vi "Get SMO HELP.vi"(8 "error in (no error)":errorcluster, 10 "Command":string, 11 "Instrument.Framework-Template in":refnum<class "Instrument.Framework-Template.lvclass">) -> (0 "error out":errorcluster, 2 "output cluster":T1, 3 "Instrument.Framework-Template out":refnum<class "Instrument.Framework-Template.lvclass">)   [LabVIEW 2019, in "Instrument.Framework-Template.lvclass"]
uses:
  Instrument.Framework-Template.lvclass
  C:/Users/patrick/Documents/GitHub/Instrument-Framework/lvsrc/Framework/Instrument/Instrument.lvclass
  <userlib>/LevyLab/Instrument Framework/Instrument/Help/typedefs/Help--cluster.ctl
  Typedefs/Instrument.Framework-Template.PublicCommands--Enum.ctl
  <userlib>/LevyLab/Instrument Framework/Instrument Types/SCPI/Instrument.SCPI.lvclass
  <userlib>/LevyLab/Instrument Framework/Instrument/Help/Help.lvclass
  <userlib>/LevyLab/Instrument Framework/Instrument/Instrument.lvclass
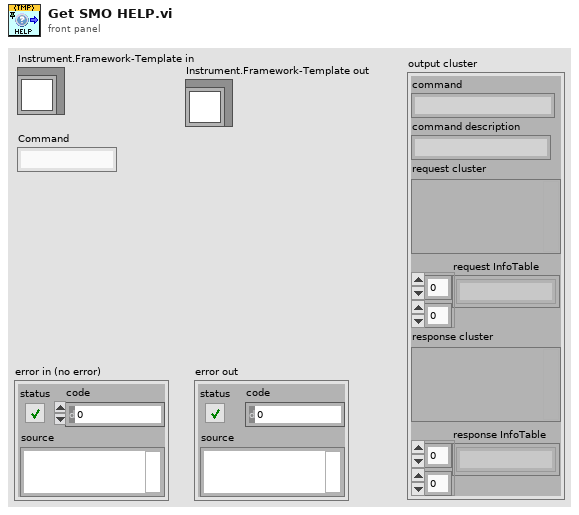
[diagram p1: front panel]
types:
  T1 = typedef "Help.lvclass/Help--cluster.ctl" = cluster{"command":string, "command description":string, "request cluster":variant, "request InfoTable":string[][], "response cluster":variant, "response InfoTable":string[][]}
  T2 = typedef "Instrument.Framework-Template.lvclass/Instrument.Framework-Template.PublicCommands--Enum.ctl" = enum16{"doSomething"}
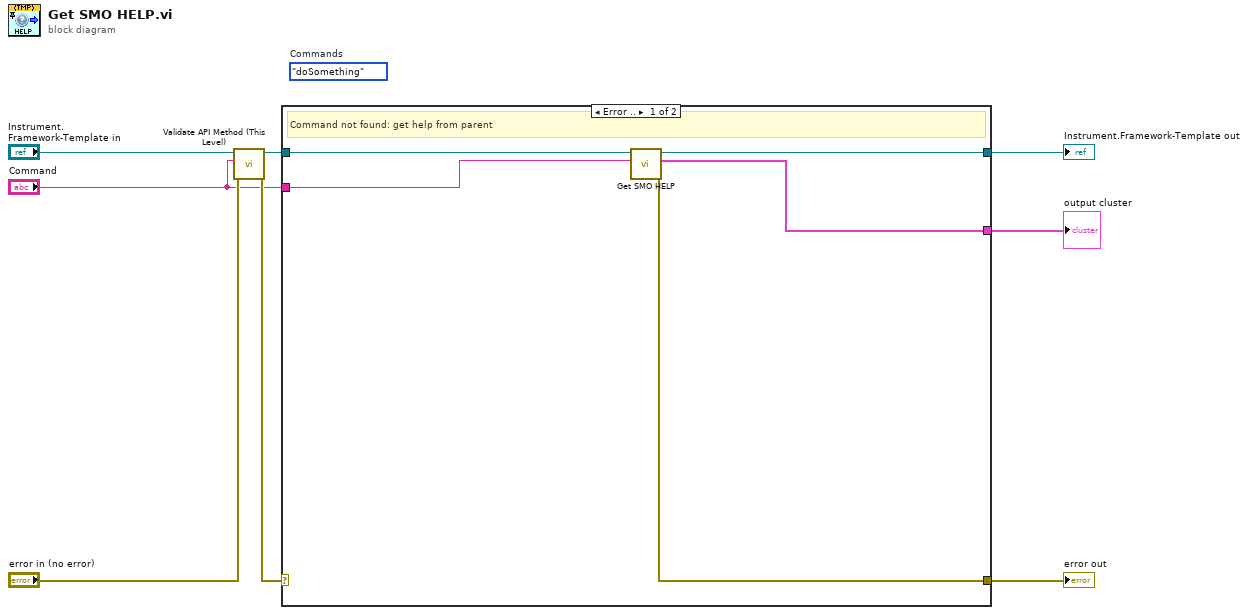
[diagram p0: block diagram]
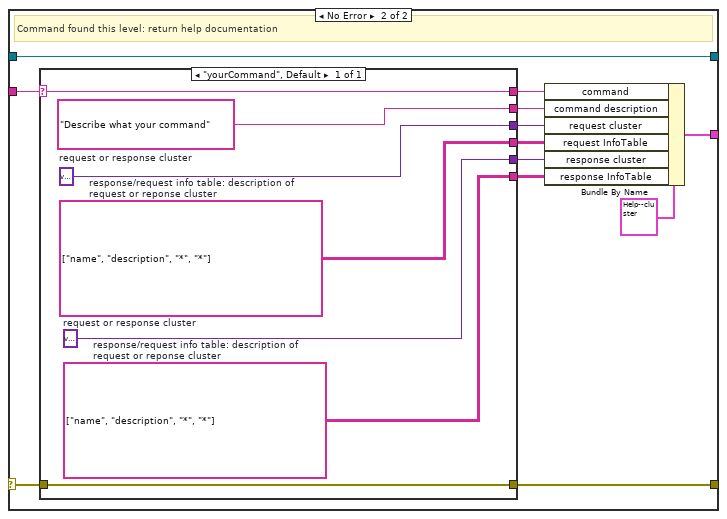
[diagram p2: hidden frame]
diagram:
  (unwired) Instrument.Framework-Template.PublicCommands--Enum."doSomething"  # Commands
  n1 = call <userlib>:"Validate API Method (This Level).vi"("error in (no error)"="error in (no error)", "Command in"="Command", "Instrument in"="Instrument.Framework-Template in") -> ("error out"=w3:errorcluster, "Instrument out"=w2:refnum<class "Instrument.Framework-Template.lvclass">)  [unwired: 6 in, 1 out]
  n2 = case shown="Error .." w3 {
    selector: w3 -> [_ w20]
    tunnel: w2 -> [w13 w25]
    tunnel: [w12 w25] -> w5
    tunnel: [w10 w19] -> w8
    tunnel: [w9 w24] -> w4
    tunnel: "Command" -> [w11 w22]
    frame Error {
      # "Command not found: get help from parent"
      n3 = call-parent "Get SMO HELP.vi"("Command"=w11, "Instrument in"=w13) -> ("error out"=w10:errorcluster, "output cluster"=w9:T1, "Instrument out"=w12:refnum<class "Instrument.Framework-Template.lvclass">)  [unwired: 7 in]
    }
    frame No Error {
      # "Command found this level: return help documentation"
      n4 = case shown="\"yourCommand\", Default" w22 {
        selector: w22 -> [w32]
        tunnel: [w32] -> w21
        tunnel: w20 -> [w31]
        tunnel: [w31] -> w19
        tunnel: ["Describe what your command"] -> w18
        tunnel: [w29] -> w17
        tunnel: [w28] -> w16
        tunnel: [w27] -> w15
        tunnel: [w26] -> w14
        frame "yourCommand", Default {
          w29 = variant  # request or response cluster
          w28 = string[][] [["name", "description"], ["*", "*"]]  # response/request info table: description of request or reponse cluster
          w27 = variant  # request or response cluster
          w26 = string[][] [["name", "description"], ["*", "*"]]  # response/request info table: description of request or reponse cluster
        }
      }
      n5 = Bundle By Name(cluster=T1 {"command"="", "command description"="", "request cluster"=variant, "request InfoTable"=[], "response cluster"=variant, "response InfoTable"=[]} ("Help"), "command"=w21, "command description"=w18, "request cluster"=w17, "request InfoTable"=w16, "response cluster"=w15, "response InfoTable"=w14) -> (w24:T1)
    }
  }
  "Instrument.Framework-Template out" <- w5
  "output cluster" <- w4
  "error out" <- w8
